vi "Test Digital Channel.vi"(8 "error in (no error)":errorcluster, 9 "Channel (0)":u32, 10 "Test Label":string, 11 "CT Common Tests in":refnum<class "CT Common Tests.lvclass">) -> (0 "error out":errorcluster, 1 "Result":string, 2 "Passed":bool, 3 "CT Common Tests out":refnum<class "CT Common Tests.lvclass">)   [LabVIEW 2015, in "CT Common Tests.lvclass"]
uses:
  CT Common Tests.lvclass
  Classes/Instruments/MIO Device/MIO Device/Class/typedefs/Read Type -- Enum.ctl
  Classes/Instruments/MIO Device/MIO Device/Class/typedefs/Channel Type -- Enum.ctl
  Classes/Instruments/MIO Device/MIO Device/Class/MIO Device.lvclass
  Classes/Application/Class/Application.lvclass
  Classes/Test Recipe/Class/Test Recipe.lvclass
  Test Class/Test Class.lvclass
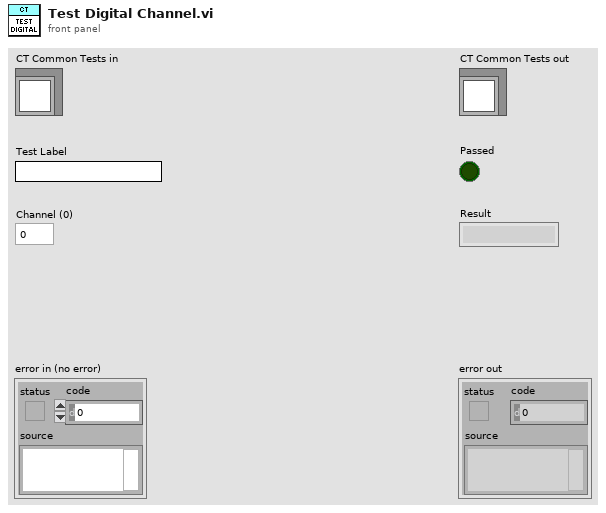
[diagram p1: front panel]
types:
  T1 = typedef "MIO Device.lvlib/MIO Device.lvclass/Channel Type -- Enum.ctl" = enum16{"Analog Input", "Analog Output", "Digital Input", "Digital Output"}
  T2 = typedef "MIO Device.lvlib/MIO Device.lvclass/Read Type -- Enum.ctl" = enum16{"Get All", "Get Latest", "Get Average"}
  T3 = typedef "Application.lvlib/App Properties.lvclass/Class Properties -- Cluster.ctl" = cluster{"UUT Info":T4[], "Test Information":refnum<vi>, "Test Complete Event":refnum<user-event>, "Shop Floor System":refnum<class "Shop Floor System.lvclass">, "Gold Board":refnum<class "Golden Board.lvclass">, "Test Recipe":refnum<class "Test Recipe.lvclass">, "Instruments":refnum<class "Instrument.lvclass">[], "Mode":T5, "Test Results":cluster{"Pass":bool[], "Fail Codes":string[]}, "Station Config":refnum<class "Station Config.lvclass">}
  T4 = typedef "Application.lvlib/App Properties.lvclass/UUT Reference -- Cluster.ctl" = cluster{"Serial Number Reference":refnum<vi>, "Status Message Reference":refnum<vi>}
  T5 = typedef "Application.lvlib/Application.lvclass/Op Mode -- Enum.ctl" = u16
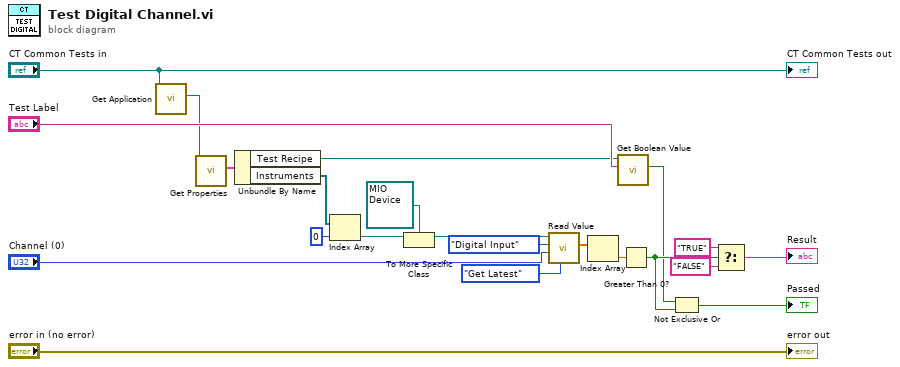
[diagram p0: block diagram]
diagram:
  n1 = call "Get Application.vi"("Test Class in"="CT Common Tests in") -> ("Application.lvlib:Application.lvclass"=w16:refnum<class "Application.lvclass">)  [unwired: 9 in, 1 out]
  n2 = call "Get Properties.vi"("Acrobat Template in"=w16) -> ("Class Properties"=w4:T3)  [unwired: 8 in, 2 out]
  n3 = Unbundle By Name(w4) -> ("Test Recipe"=w10:refnum<class "Test Recipe.lvclass">, "Instruments"=w5:refnum<class "Instrument.lvclass">[])
  n4 = Index Array(array=w5, index=0) -> (element=w6:refnum<class "Instrument.lvclass">)
  n5 = To More Specific Class(target class=refnum<class "MIO Device.lvclass"> refnum ("MIO Device.lvlib:MIO Device.lvclass"), reference=w6) -> (specific class reference=w8:refnum<class "MIO Device.lvclass">)  [unwired: 1 in, 1 out]
  n6 = call-dynamic "Read Value.vi"("Read Function (Get All)"=Read_Type_--_Enum."Get Latest", "Channel (0)"="Channel (0)", "Channel Type"=Channel_Type_--_Enum."Digital Input", "MIO Device in"=w8) -> ("First Channel"=w9:dbl[])  [unwired: 4 in, 3 out]
  n7 = Index Array(array=w9) -> (element=w11:dbl)  [unwired: 1 in]
  n8 = call "Get Boolean Value.vi"("Name"="Test Label", "Test Recipe in"=w10) -> ("Value"=w14:bool)  [unwired: 7 in, 2 out]
  n9 = Greater Than 0?(x=w11) -> (x > 0?=w15:bool)
  n10 = Not Exclusive Or(1:w15, 2:w14) -> (0:→"Passed":bool)
  n11 = Select(t="TRUE", s=w15, f="FALSE") -> (s? t:f=→"Result":string)
  "error out" <- "error in (no error)"
  "CT Common Tests out" <- "CT Common Tests in"
